vi "告警码字段定义.vi"(11 "告警代码":u16) -> (1 "故障详情":string, 2 "通用告警信息":string, 3 "字符串":string)   [LabVIEW 2016, in "斯坦道总磷.lvlib"]
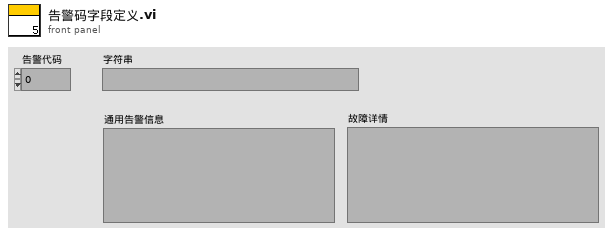
[diagram p1: front panel]
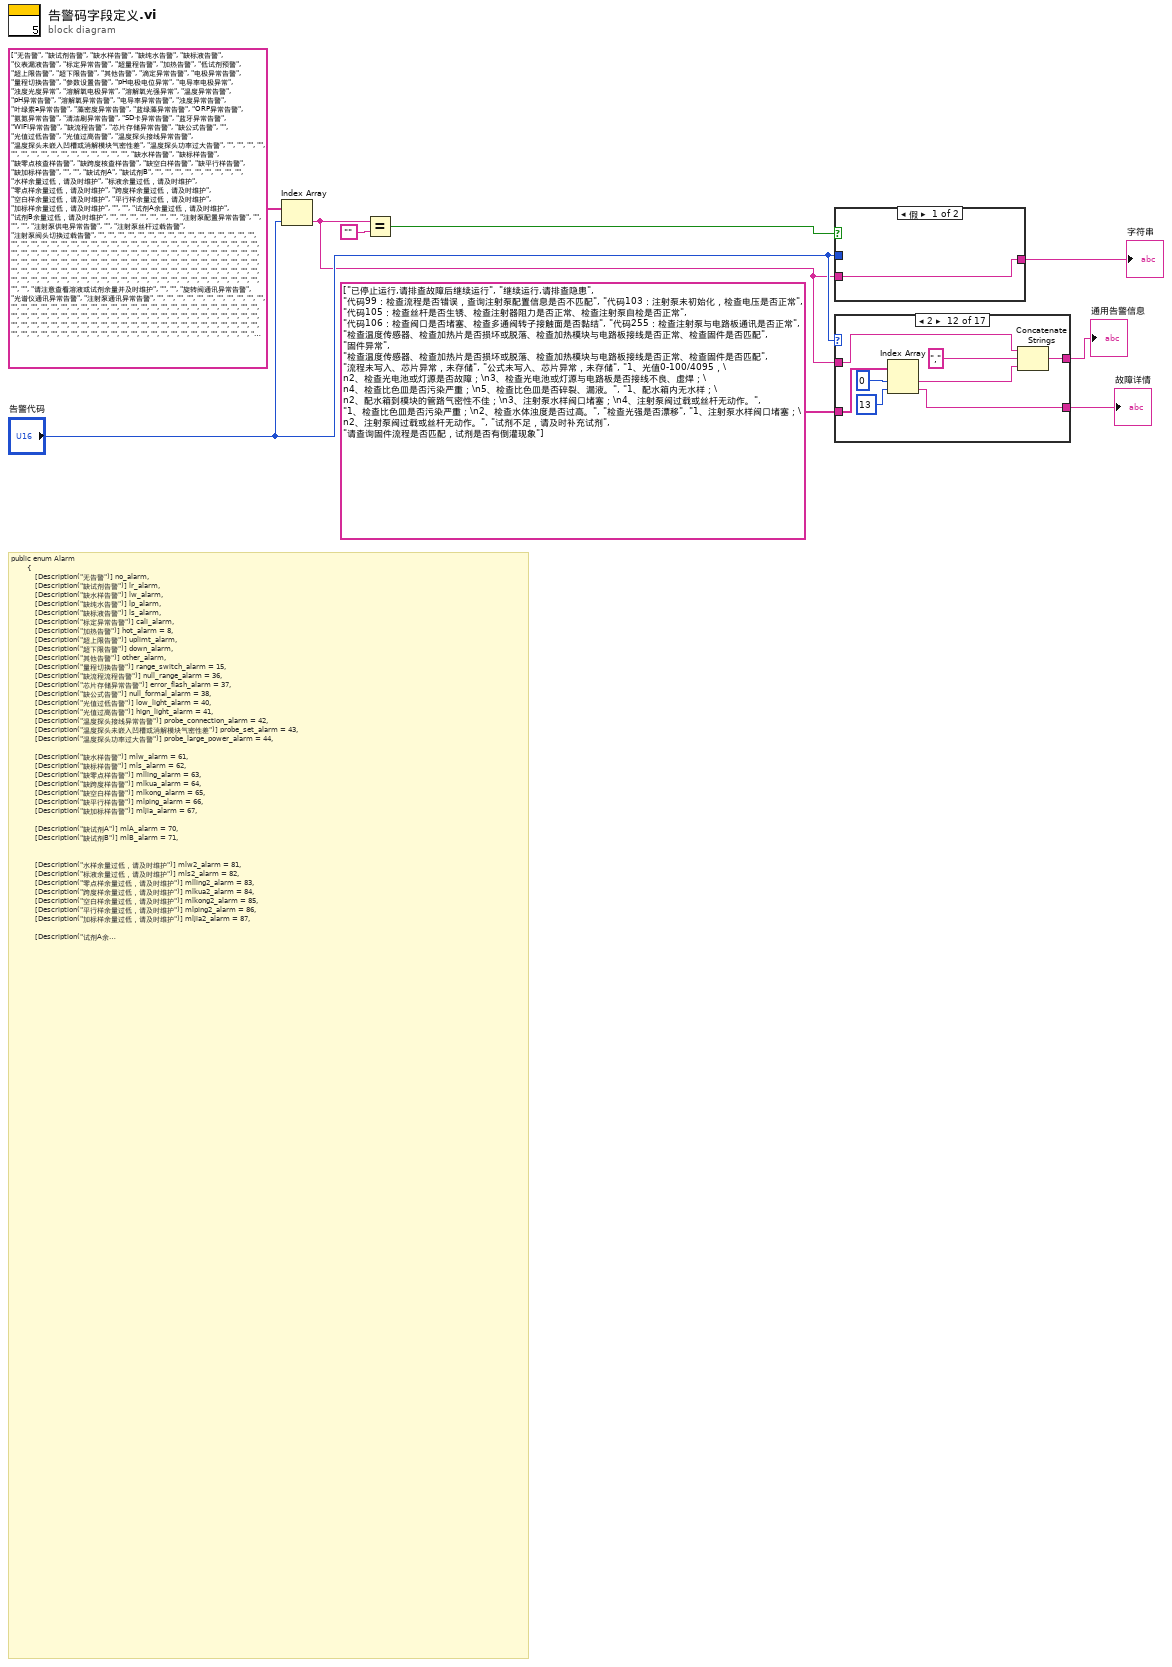
[diagram p0: block diagram]
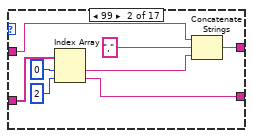
[diagram p3: hidden frame]
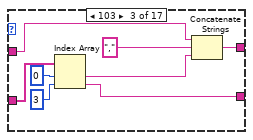
[diagram p4: hidden frame]
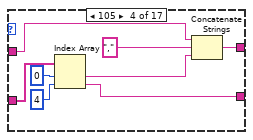
[diagram p5: hidden frame]
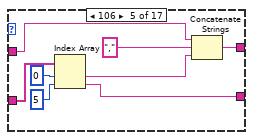
[diagram p6: hidden frame]
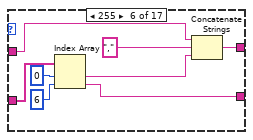
[diagram p7: hidden frame]
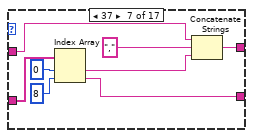
[diagram p8: hidden frame]
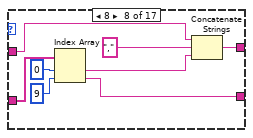
[diagram p9: hidden frame]
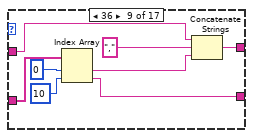
[diagram p10: hidden frame]
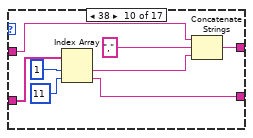
[diagram p11: hidden frame]
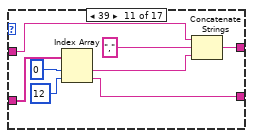
[diagram p12: hidden frame]
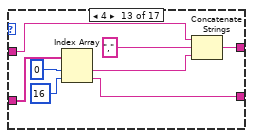
[diagram p13: hidden frame]
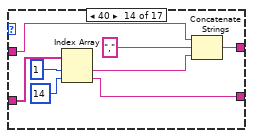
[diagram p14: hidden frame]
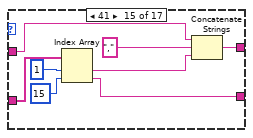
[diagram p15: hidden frame]
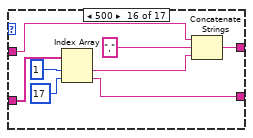
[diagram p16: hidden frame]
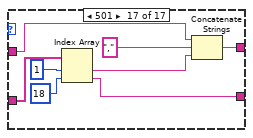
[diagram p17: hidden frame]
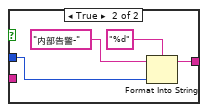
[diagram p18: hidden frame]
diagram:
  # "public enum Alarm\n        {\n            [Description(\"无告警\")] no_alarm,\n            [Description(\"缺试剂告警\")] lr_alarm,\n            [Description(\"缺水样告警\")] lw_alarm,\n            [Description(\"缺纯水告警\")] lp_alarm,\n            [Description(\"缺标液告警\")] ls_alarm,\n            [Description(\"标定异常告警\")] cali_alarm,\n            [Description(\"加热告警\")] hot_alarm = 8,\n            [Description(\"超上限告警\")] uplimt_alarm,\n            [Description(\"超下限告警\")] down_alarm,\n            [Description(\"其他告警\")] other_alarm,\n            [Description(\"量程切换告警\")] range_switch_alarm = 15,\n            [Description(\"缺流程流程告警\")] null_range_alarm = 36,\n            [Description(\"芯片存储异常告警\")] error_flash_alarm = 37,\n            [Description(\"缺公式告警\")] null_formal_alarm = 38,\n            [Description(\"光值过低告警\")] low_light_alarm = 40,\n            [Description(\"光值过高告警\")] hign_light_alarm = 41,\n            [Description(\"温度探头接线异常告警\")] probe_connection_alarm = 42,\n            [Description(\"温度探头未嵌入凹槽或消解模块气密性差\")] probe_set_alarm = 43,\n            [Description(\"温度探头功率过大告警\")] probe_large_power_alarm = 44,\n\n            [Description(\"缺水样告警\")] mlw_alarm = 61,\n            [Description(\"缺标样告警\")] mls_alarm = 62,\n            [Description(\"缺零点样告警\")] mlling_alarm = 63,\n            [Description(\"缺跨度样告警\")] mlkua_alarm = 64,\n            [Description(\"缺空白样告警\")] mlkong_alarm = 65,\n            [Description(\"缺平行样告警\")] mlping_alarm = 66,\n            [Description(\"缺加标样告警\")] mljia_alarm = 67,\n\n            [Description(\"缺试剂A\")] mlA_alarm = 70,\n            [Description(\"缺试剂B\")] mlB_alarm = 71,\n\n\n            [Description(\"水样余量过低，请及时维护\")] mlw2_alarm = 81,\n            [Description(\"标液余量过低，请及时维护\")] mls2_alarm = 82,\n            [Description(\"零点样余量过低，请及时维护\")] mlling2_alarm = 83,\n            [Description(\"跨度样余量过低，请及时维护\")] mlkua2_alarm = 84,\n            [Description(\"空白样余量过低，请及时维护\")] mlkong2_alarm = 85,\n            [Description(\"平行样余量过低，请及时维护\")] mlping2_alarm = 86,\n            [Description(\"加标样余量过低，请及时维护\")] mljia2_alarm = 87,\n\n            [Description(\"试剂A余量过低，请及时维护\")] mlA2_alarm = 90,\n            [Description(\"试剂B余量过低，请及时维护\")] mlB2_alarm = 91,\n\n\n            [Description(\"注射泵供电告警\")] pump_Not_Initialized_alarm = 103,\n            [Description(\"注释泵丝杆过载过载告警\")] pump_Plunger_Overload_alarm = 105,\n            [Description(\"注释泵阀头切换过载告警\")] pump_Valve_Overload_alarm = 106,\n            [Description(\"注射泵配置异常告警\")] pump_Valve_Config_alarm = 99,\n            [Description(\"请注意查看溶液或试剂余量并及时维护\")] reagentRemaid_alarm = 250,\n            [Description(\"旋转阀通信异常告警\")] valve_commuication_alarm = 253,\n            [Description(\"光谱仪通信异常告警\")] spec_commuication_alarm = 254,\n            [Description(\"注射泵通信异常告警\")] pump_commuication_alarm = 255,\n        }\n        public enum Error\n        {\n            [Description(\"无故障\")] no_error,\n            [Description(\"注射泵故障\")] pump_error,\n            [Description(\"加热故障\")] hot_error,\n            [Description(\"旋转阀故障\")] value_error,\n\n            [Description(\"光值过低故障\")] low_light_error = 38,\n            [Description(\"光路系统故障\")] error_light_error = 39,\n        }"
  n1 = Index Array(array=string[] ["无告警", "缺试剂告警", "缺水样告警", "缺纯水告警", "缺标液告警", "仪表漏液告警", "标定异常告警", "超量程告警", "加热告警", "低试剂预警", "超上限告警", "超下限告警", "其他告警", "滴定异常告警", "电极异常告警", "量程切换告警", "参数设置告警", "pH电极电位异常", "电导率电极异常", "浊度光度异常", "溶解氧电极异常", "溶解氧光强异常", "温度异常告警", "pH异常告警", "溶解氧异常告警", "电导率异常告警", "浊度异常告警", "叶绿素a异常告警", "藻密度异常告警", "蓝绿藻异常告警", "ORP异常告警", "氨氮异常告警", "清洁刷异常告警", "SD卡异常告警", "蓝牙异常告警", "WIFI异常告警", "缺流程告警", "芯片存储异常告警", "缺公式告警", "", "光值过低告警", "光值过高告警", "温度探头接线异常告警", "温度探头未嵌入凹槽或消解模块气密性差", "温度探头功率过大告警", "", "", "", "", "", "", "", "", "", "", "", "", "", "", "", "", "缺水样告警", "缺标样告警", "缺零点核查样告警", "缺跨度核查样告警", "缺空白样告警", "缺平行样告警", "缺加标样告警", "", "", "缺试剂A", "缺试剂B", "", "", "", "", "", "", "", "", "", "水样余量过低，请及时维护", "标液余量过低，请及时维护", "零点样余量过低，请及时维护", "跨度样余量过低，请及时维护", "空白样余量过低，请及时维护", "平行样余量过低，请及时维护", "加标样余量过低，请及时维护", "", "", "试剂A余量过低，请及时维护", "试剂B余量过低，请及时维护", "", "", "", "", "", "", "", "注射泵配置异常告警", "", "", "", "注射泵供电异常告警", "", "注射泵丝杆过载告警", "注射泵阀头切换过载告警", "", "", "", "", "", "", "", "", "", "", "", "", "", "", "", "", "", "", "", "", "", "", "", "", "", "", "", "", "", "", "", "", "", "", "", "", "", "", "", "", "", "", "", "", "", "", "", "", "", "", "", "", "", "", "", "", "", "", "", "", "", "", "", "", "", "", "", "", "", "", "", "", "", "", "", "", "", "", "", "", "", "", "", "", "", "", "", "", "", "", "", "", "", "", "", "", "", "", "", "", "", "", "", "", "", "", "", "", "", "", "", "", "", "", "", "", "", "", "", "", "", "", "", "", "", "", "", "", "", "", "", "", "", "", "", "", "", "", "", "", "", "", "", "请注意查看溶液或试剂余量并及时维护", "", "", "旋转阀通讯异常告警", "光谱仪通讯异常告警", "注射泵通讯异常告警", "", "", "", "", "", "", "", "", "", "", "", "", "", "", "", "", "", "", "", "", "", "", "", "", "", "", "", "", "", "", "", "", "", "", "", "", "", "", "", "", "", "", "", "", "", "", "", "", "", "", "", "", "", "", "", "", "", "", "", "", "", "", "", "", "", "", "", "", "", "", "", "", "", "", "", "", "", "", "", "", "", "", "", "", "", "", "", "", "", "", "", "", "", "", "", "", "", "", "", "", "", "", "", "", "", "", "", "", "", "", "", "", "", "", "", "", "", "", "", "", "", "", "", "", "", "", "", "", "", "", "", "", "", "", "", "", "", "", "", "", "", "", "", "", "", "", "", "", "", "", "", "", "", "", "", "", "", "", "", "", "", "", "", "", "", "", "", "", "", "", "", "", "", "", "", "", "", "", "", "", "", "", "", "", "", "", "", "", "", "", "", "", "", "", "", "", "", "", "", "", "", "", "", "", "", "", "", "", "", "", "", "", "", "", "", "", "", "", "", "", "", "", "", "", "", "", "", "", "", "", "", "", "", "", "", "", "", "", "", "", "", "", "", "", "试剂不足", "试剂余量检测异常"], index="告警代码") -> (element=w5:string)
  n2 = Equal?(x=w5, y="") -> (x = y?=w8:bool)
  n3 = case shown="假" w8 {
    tunnel: [w10 w12] -> w7
    tunnel: w5 -> [w10 _]
    tunnel: "告警代码" -> [_ w11]
    frame False {
    }
    frame True {
      n4 = Format Into String(format string="%d" ("格式字符串"), initial string="内部告警-" ("工作状态"), w11) -> (resulting string=w12:string)  [unwired: 1 in, 1 out]
    }
  }
  "字符串" <- w7
  n5 = case shown="2" "告警代码" {
    tunnel: string[] ["已停止运行,请排查故障后继续运行", "继续运行,请排查隐患", "代码99：检查流程是否错误，查询注射泵配置信息是否不匹配", "代码103：注射泵未初始化，检查电压是否正常", "代码105：检查丝杆是否生锈、检查注射器阻力是否正常、检查注射泵自检是否正常", "代码106：检查阀口是否堵塞、检查多通阀转子接触面是否黏结", "代码255：检查注射泵与电路板通讯是否正常", "检查温度传感器、检查加热片是否损坏或脱落、检查加热模块与电路板接线是否正常、检查固件是否匹配", "固件异常", "检查温度传感器、检查加热片是否损坏或脱落、检查加热模块与电路板接线是否正常、检查固件是否匹配", "流程未写入、芯片异常，未存储", "公式未写入、芯片异常，未存储", "1、光值0-100/4095，\n2、检查光电池或灯源是否故障；\n3、检查光电池或灯源与电路板是否接线不良、虚焊；\n4、检查比色皿是否污染严重；\n5、检查比色皿是否碎裂、漏液。", "1、配水箱内无水样；\n2、配水箱到模块的管路气密性不佳；\n3、注射泵水样阀口堵塞；\n4、注射泵阀过载或丝杆无动作。", "1、检查比色皿是否污染严重；\n2、检查水体浊度是否过高。", "检查光强是否漂移", "1、注射泵水样阀口堵塞；\n2、注射泵阀过载或丝杆无动作。", "试剂不足，请及时补充试剂", "请查询固件流程是否匹配，试剂是否有倒灌现象"] -> [_ w23 w31 w39 w47 w55 w63 w71 w79 w87 w95 w103 w111 w119 w127 w135 w143]
    tunnel: [w15 w18 w26 w34 w42 w50 w58 w66 w74 w82 w90 w98 w106 w114 w122 w130 w138] -> w3
    tunnel: [_ w19 w27 w35 w43 w51 w59 w67 w75 w83 w91 w99 w107 w115 w123 w131 w139] -> w2
    tunnel: w5 -> [w15 w17 w25 w33 w41 w49 w57 w65 w73 w81 w89 w97 w105 w113 w121 w129 w137]
    frame 0, Default {
    }
    frame 99 {
      n6 = Index Array(array=w23, index #1=0 ("索引"), index #2=2 ("索引")) -> (element #1=w21:string, element #2=w19:string)
      n7 = Concatenate Strings(w17, "," ("字符串"), w21) -> (w18:string)
    }
    frame 103 {
      n8 = Index Array(array=w31, index #1=0 ("索引"), index #2=3 ("索引")) -> (element #1=w29:string, element #2=w27:string)
      n9 = Concatenate Strings(w25, "," ("字符串"), w29) -> (w26:string)
    }
    frame 105 {
      n10 = Index Array(array=w39, index #1=0 ("索引"), index #2=4 ("索引")) -> (element #1=w37:string, element #2=w35:string)
      n11 = Concatenate Strings(w33, "," ("字符串"), w37) -> (w34:string)
    }
    frame 106 {
      n12 = Index Array(array=w47, index #1=0 ("索引"), index #2=5 ("索引")) -> (element #1=w45:string, element #2=w43:string)
      n13 = Concatenate Strings(w41, "," ("字符串"), w45) -> (w42:string)
    }
    frame 255 {
      n14 = Index Array(array=w55, index #1=0 ("索引"), index #2=6 ("索引")) -> (element #1=w53:string, element #2=w51:string)
      n15 = Concatenate Strings(w49, "," ("字符串"), w53) -> (w50:string)
    }
    frame 37 {
      n16 = Index Array(array=w63, index #1=0 ("索引"), index #2=8 ("索引")) -> (element #1=w61:string, element #2=w59:string)
      n17 = Concatenate Strings(w57, "," ("字符串"), w61) -> (w58:string)
    }
    frame 8 {
      n18 = Index Array(array=w71, index #1=0 ("索引"), index #2=9 ("索引")) -> (element #1=w69:string, element #2=w67:string)
      n19 = Concatenate Strings(w65, "," ("字符串"), w69) -> (w66:string)
    }
    frame 36 {
      n20 = Index Array(array=w79, index #1=0 ("索引"), index #2=10 ("索引")) -> (element #1=w77:string, element #2=w75:string)
      n21 = Concatenate Strings(w73, "," ("字符串"), w77) -> (w74:string)
    }
    frame 38 {
      n22 = Index Array(array=w87, index #1=1 ("索引"), index #2=11 ("索引")) -> (element #1=w85:string, element #2=w83:string)
      n23 = Concatenate Strings(w81, "," ("字符串"), w85) -> (w82:string)
    }
    frame 39 {
      n24 = Index Array(array=w95, index #1=0 ("索引"), index #2=12 ("索引")) -> (element #1=w93:string, element #2=w91:string)
      n25 = Concatenate Strings(w89, "," ("字符串"), w93) -> (w90:string)
    }
    frame 2 {
      n26 = Index Array(array=w103, index #1=0 ("索引"), index #2=13 ("索引")) -> (element #1=w101:string, element #2=w99:string)
      n27 = Concatenate Strings(w97, "," ("字符串"), w101) -> (w98:string)
    }
    frame 4 {
      n28 = Index Array(array=w111, index #1=0 ("索引"), index #2=16 ("索引")) -> (element #1=w109:string, element #2=w107:string)
      n29 = Concatenate Strings(w105, "," ("字符串"), w109) -> (w106:string)
    }
    frame 40 {
      n30 = Index Array(array=w119, index #1=1 ("索引"), index #2=14 ("索引")) -> (element #1=w117:string, element #2=w115:string)
      n31 = Concatenate Strings(w113, "," ("字符串"), w117) -> (w114:string)
    }
    frame 41 {
      n32 = Index Array(array=w127, index #1=1 ("索引"), index #2=15 ("索引")) -> (element #1=w125:string, element #2=w123:string)
      n33 = Concatenate Strings(w121, "," ("字符串"), w125) -> (w122:string)
    }
    frame 500 {
      n34 = Index Array(array=w135, index #1=1 ("索引"), index #2=17 ("索引")) -> (element #1=w133:string, element #2=w131:string)
      n35 = Concatenate Strings(w129, "," ("字符串"), w133) -> (w130:string)
    }
    frame 501 {
      n36 = Index Array(array=w143, index #1=1 ("索引"), index #2=18 ("索引")) -> (element #1=w141:string, element #2=w139:string)
      n37 = Concatenate Strings(w137, "," ("字符串"), w141) -> (w138:string)
    }
  }
  "通用告警信息" <- w3
  "故障详情" <- w2
